vi "Omni (SubVI).vi"(8 "Vp":dbl, 9 "Vy":dbl, 10 "Vx":dbl) -> (0 "Back_Right":dbl, 1 "Back_Left":dbl, 2 "Front_Right":dbl, 3 "Front_Left":dbl)   [LabVIEW 2017]
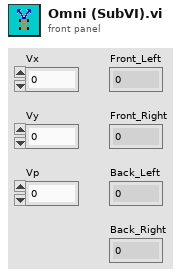
[diagram p1: front panel]
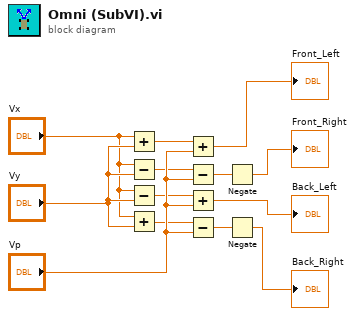
[diagram p0: block diagram]
diagram:
  n1 = Add(x="Vx", y="Vy") -> (x+y=w6:dbl)
  n2 = Subtract(x="Vx", y="Vy") -> (x-y=w7:dbl)
  n3 = Subtract(x="Vx", y="Vy") -> (x-y=w8:dbl)
  n4 = Add(x="Vx", y="Vy") -> (x+y=w9:dbl)
  n5 = Add(x=w6, y="Vp") -> (x+y=→"Front_Left":dbl)
  n6 = Subtract(x=w7, y="Vp") -> (x-y=w12:dbl)
  n7 = Add(x=w8, y="Vp") -> (x+y=→"Back_Left":dbl)
  n8 = Subtract(x=w9, y="Vp") -> (x-y=w2:dbl)
  n9 = Negate(x=w12) -> (-x=→"Front_Right":dbl)
  n10 = Negate(x=w2) -> (-x=→"Back_Right":dbl)
